vi "thermal_noise_calculator.vi"() -> ()   [LabVIEW 2021]
panel:
  in  "Numeric":dbl
  in  "constant":dbl
  in  "constant":dbl
  out "Johnson Nyquist noise voltage (V)":dbl
  in  "Bandwidth (Hz)":dbl
  in  "Resistance (Ohm)":dbl
  in  "Temperature (K)":dbl
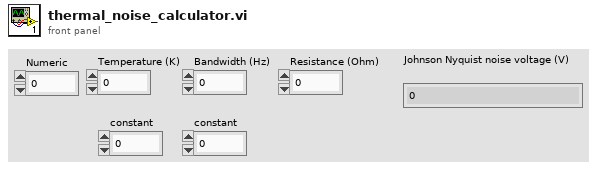
[diagram p1: front panel]
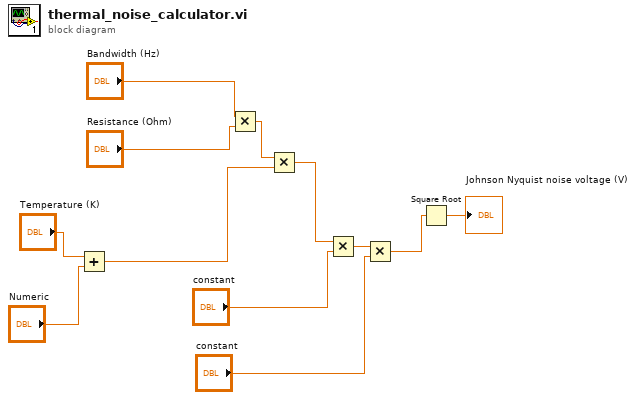
[diagram p0: block diagram]
diagram:
  n1 = Add(x="Temperature (K)", y="Numeric") -> (x+y=w2:dbl)
  n2 = Multiply(x="Bandwidth (Hz)", y="Resistance (Ohm)") -> (x*y=w10:dbl)
  n3 = Multiply(x=w10, y=w2) -> (x*y=w8:dbl)
  n4 = Multiply(x=w8, y="constant") -> (x*y=w6:dbl)
  n5 = Multiply(x=w6, y="constant") -> (x*y=w5:dbl)
  n6 = Square Root(x=w5) -> (sqrt(x)=→"Johnson Nyquist noise voltage (V)":dbl)
